vi "ReadMQTTandUpdateFPGA.vi"(8 "error in (no error)":errorcluster, 9 "timeout ms (25000)":i32=25000, 10 "FPGA VI Reference":T1, 11 "MQTT":refnum<k5>) -> (0 "error out":errorcluster)   [LabVIEW 2024]
uses:
  FPGA VI Ref.ctl
  <vilib>/Utility/error.llb/Error Cluster From Error Code.vi
  <vilib>/rvi/errors/niLvFpgaAdjustHostInterfaceError.vi
  <vilib>/rvi/interface/nirviReadWriteControl/nirviReadWriteControl.xnode
  LVMQTT-master/MQTT_Functions.lvlib
  NiFpgaLv.dll
  <vilib>/rvi/interface/Simulation/niFpgaSimulationCallBeginRW.vi
panel:
  out "Message":string
  out "value":T2
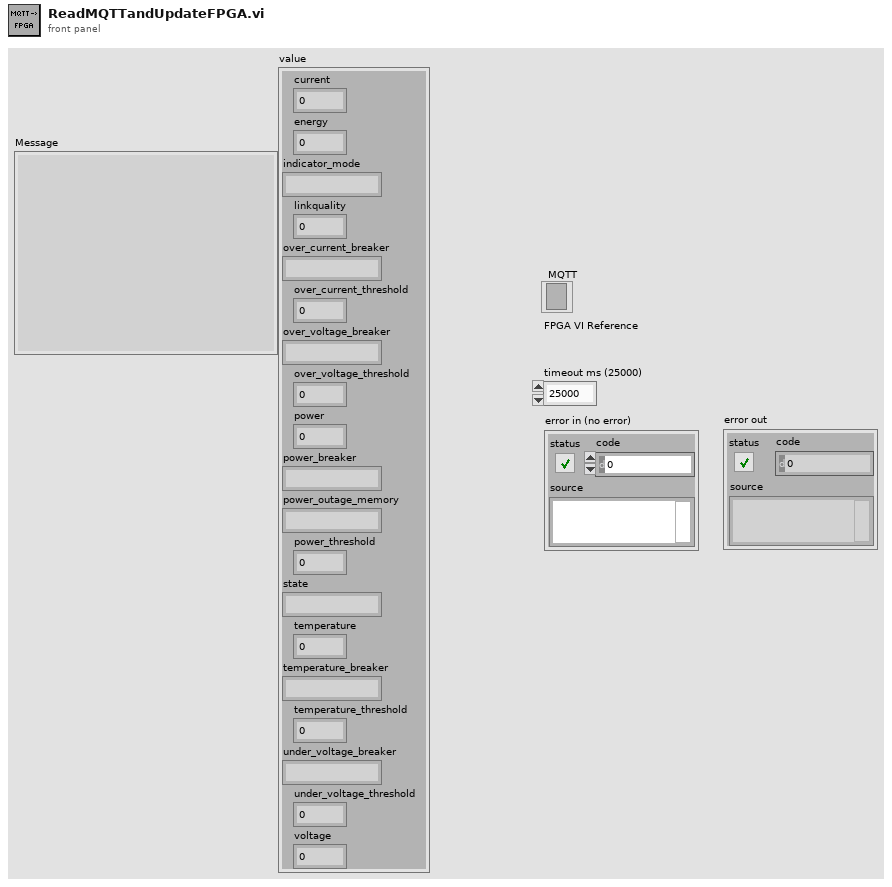
[diagram p1: front panel]
types:
  T1 = typedef "FPGA VI Ref.ctl" = refnum<k20>
  T2 = cluster{"current":dbl, "energy":dbl, "indicator_mode":string, "linkquality":i32, "over_current_breaker":string, "over_current_threshold":dbl, "over_voltage_breaker":string, "over_voltage_threshold":dbl, "power":dbl, "power_breaker":string, "power_outage_memory":string, "power_threshold":dbl, "state":string, "temperature":dbl, "temperature_breaker":string, "temperature_threshold":dbl, "under_voltage_breaker":string, "under_voltage_threshold":dbl, "voltage":dbl}
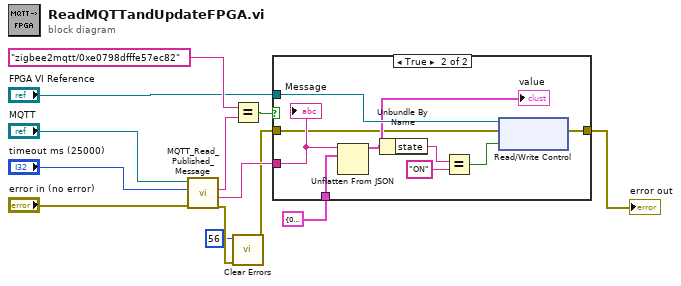
[diagram p0: block diagram]
diagram:
  n1 = call "MQTT_Read_Published_Message.vi"("error in (no error)"="error in (no error)", "timeout ms (25000)"="timeout ms (25000)", "connection ID"="MQTT") -> ("error out"=w4:errorcluster, "Message"=w13:string, "Topic Name"=w12:string)  [unwired: 3 in, 3 out]
  n2 = Equal?(x="zigbee2mqtt/0xe0798dfffe57ec82" ("Topic"), y=w12) -> (x = y?=w11:bool)
  n3 = call <vilib>:"Clear Errors.vi"("error in (no error)"=w4, "specific error code to clear (0: all)"=56) -> ("error out"=w3:errorcluster)  [unwired: 4 in, 1 out]
  n4 = case shown="True" w11 {
    tunnel: w13 -> [_ w23]
    tunnel: "FPGA VI Reference" -> [_ w22]
    tunnel: T2 {"current"=0.0, "energy"=0.68, "indicator_mode"="off/on", "linkquality"=69, "over_current_breaker"="OFF", "over_current_threshold"=0.0, "over_voltage_breaker"="OFF", "over_voltage_threshold"=0.0, "power"=0.0, "power_breaker"="OFF", "power_outage_memory"="off", "power_threshold"=13.0, "state"="OFF", "temperature"=22.28, "temperature_breaker"="OFF", "temperature_threshold"=100.0, "under_voltage_breaker"="OFF", "under_voltage_threshold"=0.0, "voltage"=238.0} ("value 2") -> [_ w17]
    tunnel: w3 -> [w14 w16]
    tunnel: [w14 w15] -> w5
    frame False {
    }
    frame True {
      n5 = Unflatten From JSON(JSON string=w23, type and defaults=w17) -> (value=w18:T2)  [unwired: 5 in, 1 out]
      "value" <- w18
      n6 = Unbundle By Name(w18) -> ("state"=w21:string)
      n7 = Equal?(x=w21, y="ON") -> (x = y?=w19:bool)
      n8 = xnode "Read/Write Control"("FPGA VI Reference In"=w22, "error in"=w16, "Kiuas LED"=w19) -> ("error out"=w15:errorcluster)  [unwired: 1 out]
      "Message" <- w23
    }
  }
  "error out" <- w5
